vi "Ex2.vi"() -> ()   [LabVIEW 2016]
uses:
  <vilib>/DAQmx/write.llb/DAQmx Write (Analog Wfm 1Chan NSamp).vi
  <vilib>/DAQmx/create/channels.llb/DAQmx Create Channel (AO-Voltage-Basic).vi
  <vilib>/DAQmx/configure/timing.llb/DAQmx Timing (Sample Clock).vi
  <vilib>/DAQmx/miscellaneous.llb/DAQmx Fill In Error Info.vi
  <vilib>/measure/NI_MABase.lvlib
panel:
  out "웨이브폼 그래프":waveform(dbl)(graph)
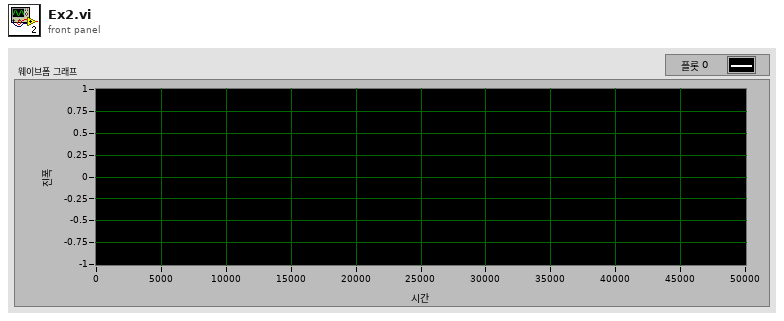
[diagram p1: front panel]
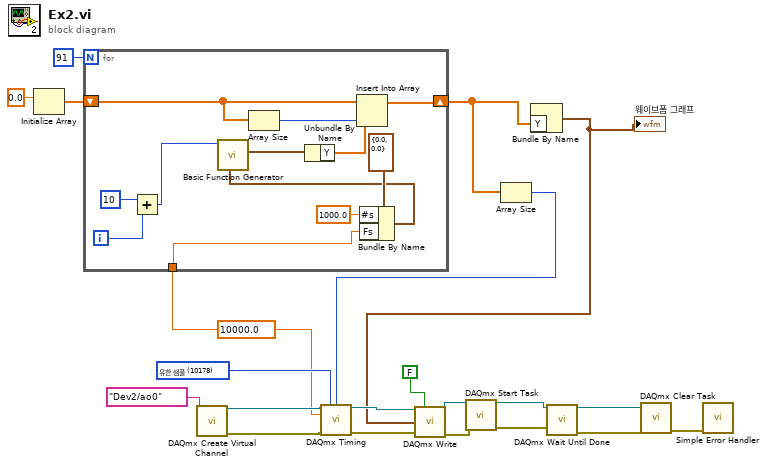
[diagram p0: block diagram]
diagram:
  w5 = 10000.0 ("rate")
  w10 = 10178 items=["유한 샘플"=10178, "연속 샘플"=10123, "하드웨어 타이밍에 의한 단일 포인트"=12522] ("sample mode")
  n1 = Initialize Array(0.0 ("원소")) -> (w14:dbl[])  [unwired: 1 in]
  n2 = for {
    N: 91 -> [_]
    shift-right: [w28] -> w11
    shift-left: w14 -> [w31]
    tunnel: w5 -> [w25]
    i -> [w33]
    n3 = Add(x=10, y=w33) -> (x+y=w26:i32)
    n4 = Array Size(array=w31) -> (size(s)=w30:i32)
    n5 = Bundle By Name(cluster=cluster{"Fs":dbl, "#s":dbl} {"Fs"=0.0, "#s"=0.0} ("sampling info"), "#s"=1000.0, "Fs"=w25) -> (w23:cluster{"Fs":dbl, "#s":dbl})
    n6 = call <vilib>:"Basic Function Generator.vi"("sampling info"=w23, "frequency"=w26) -> ("signal out"=w27:waveform(dbl))  [unwired: 7 in, 2 out]
    n7 = Unbundle By Name(w27) -> ("Y"=w29:dbl[])
    n8 = Insert Into Array(array=w31, index=w30, new element=w29) -> (w28:dbl[])
  }
  n9 = call-poly <vilib>:"DAQmx Create Virtual Channel.vi"("physical channels"=tag "Dev2/ao0") -> ("task out"=w21:refnum<k21>, "error out"=w20:errorcluster)  [unwired: 13 in]
  n10 = Array Size(array=w11) -> (size(s)=w9:i32)
  n11 = call-poly <vilib>:"DAQmx Timing.vi"("task/channels in"=w21, "sample mode"=w10, "samples per channel"=w9, "rate"=w5, "error in"=w20) -> ("task out"=w19:refnum<k21>, "error out"=w8:errorcluster)  [unwired: 9 in]
  n12 = Bundle By Name("Y"=w11) -> (w13:waveform(dbl))  [unwired: 1 in]
  "웨이브폼 그래프" <- w13
  n13 = call-poly <vilib>:"DAQmx Write.vi"("task/channels in"=w19, "auto start"=FALSE, "data"=w13, "error in"=w8) -> ("task out"=w16:refnum<k21>, "error out"=w7:errorcluster)  [unwired: 9 in, 1 out]
  n14 = call <vilib>:"DAQmx Start Task.vi"("task/channels in"=w16, "error in"=w7) -> ("task out"=w4:refnum<k21>, "error out"=w2:errorcluster)  [unwired: 12 in]
  n15 = call <vilib>:"DAQmx Wait Until Done.vi"("task/channels in"=w4, "error in"=w2) -> ("task out"=w3:refnum<k21>, "error out"=w1:errorcluster)  [unwired: 12 in]
  n16 = call <vilib>:"DAQmx Clear Task.vi"("task in"=w3, "error in"=w1) -> ("error out"=w18:errorcluster)  [unwired: 13 in]
  n17 = call <vilib>:"Simple Error Handler.vi"("error in (no error)"=w18) -> ()  [unwired: 4 in, 5 out]
